vi "SaveExcel.vi"(9 "Array 2":string[][](array[string])=[["Voltaje", "Corriente"]], 10 "Guardar en:":path, 11 "Array":dbl[][](array[numeric])) -> ()   [LabVIEW 2017]
uses:
  <vilib>/addons/_office/excel.llb/Excel Easy Table (str).vi
  <vilib>/addons/_office/excel.llb/Excel Easy Table (num).vi
  <vilib>/Utility/NIReport.llb/NI_report.lvclass
  <vilib>/addons/_office/NI_ReportGenerationToolkit.lvlib
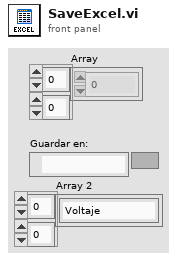
[diagram p1: front panel]
types:
  T1 = enum16{"Standard Report", "HTML", "Word", "Excel"}
  T2 = enum16{"maximized", "minimized", "normal", "no change"}
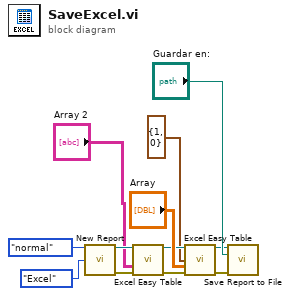
[diagram p0: block diagram]
diagram:
  n1 = call <vilib>:"New Report.vi"("window state (normal)"=T2."normal", "report type"=T1."Excel") -> ("report out"=w6:refnum<class "NI_report.lvclass">, "error out"=w5:errorcluster)  [unwired: 12 in]
  n2 = call-poly <vilib>:"Excel Easy Table.vi"("report in"=w6, "text data"="Array 2", "error in (no error)"=w5) -> ("report out"=w4:refnum<class "NI_report.lvclass">, "error out"=w3:errorcluster)  [unwired: 8 in, 3 out]
  n3 = call-poly <vilib>:"Excel Easy Table.vi"("report in"=w4, "start (0, 0)"=cluster{"row":i32, "column":i32} {"row"=1, "column"=0}, "text data"="Array", "error in (no error)"=w3) -> ("report out"=w7:refnum<class "NI_report.lvclass">, "error out"=w8:errorcluster)  [unwired: 7 in, 3 out]
  n4 = call-dynamic "Save Report to File.vi"("report in"=w7, "report file path"="Guardar en:", "error in (no error)"=w8) -> ()  [unwired: 11 in, 2 out]
